vi "Extract maximum.vi"(8 "error in (no error)":errorcluster, 11 "Image in":T1) -> (0 "error out":errorcluster, 1 "Max value":dbl, 2 "y translation":dbl, 3 "x translation":dbl)   [LabVIEW 2012]
uses:
  <vilib>/vision/Image Controls.llb/IMAQ Image.ctl
  <vilib>/vision/NI_Vision_Development_Module.lvlib
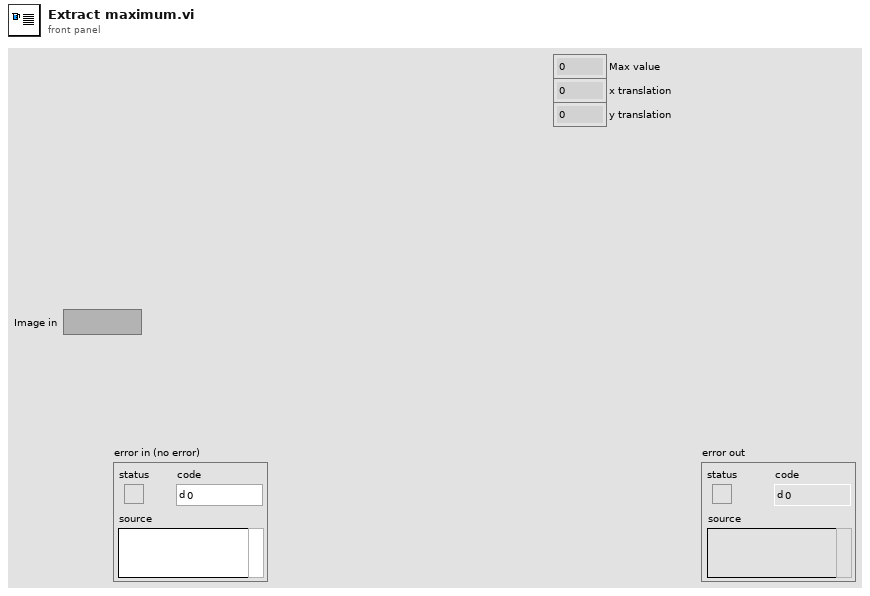
[diagram p1: front panel]
types:
  T1 = typedef "IMAQ Image.ctl" = refnum<image>
  T2 = cluster{"Mean Value":sgl, "Standard Variation":sgl, "Minimal Value":sgl, "Maximal Value":sgl, "Area (calibrated)":sgl, "Area (pixels)":u32, "%":sgl, "Calibration Valid":bool}
  T3 = cluster{"Area":dbl, "Number of Holes":dbl, "Bounding Rect":cluster{"Left":dbl, "Top":dbl, "Right":dbl, "Bottom":dbl}, "Center of Mass":cluster{"X":dbl, "Y":dbl}, "Orientation":dbl, "Dimensions":cluster{"Width":dbl, "Height":dbl}}[]
  T4 = cluster{"Area":dbl, "Number of Holes":dbl, "Bounding Rect":cluster{"Left":dbl, "Top":dbl, "Right":dbl, "Bottom":dbl}, "Center of Mass":cluster{"X":dbl, "Y":dbl}, "Orientation":dbl, "Dimensions":cluster{"Width":dbl, "Height":dbl}}
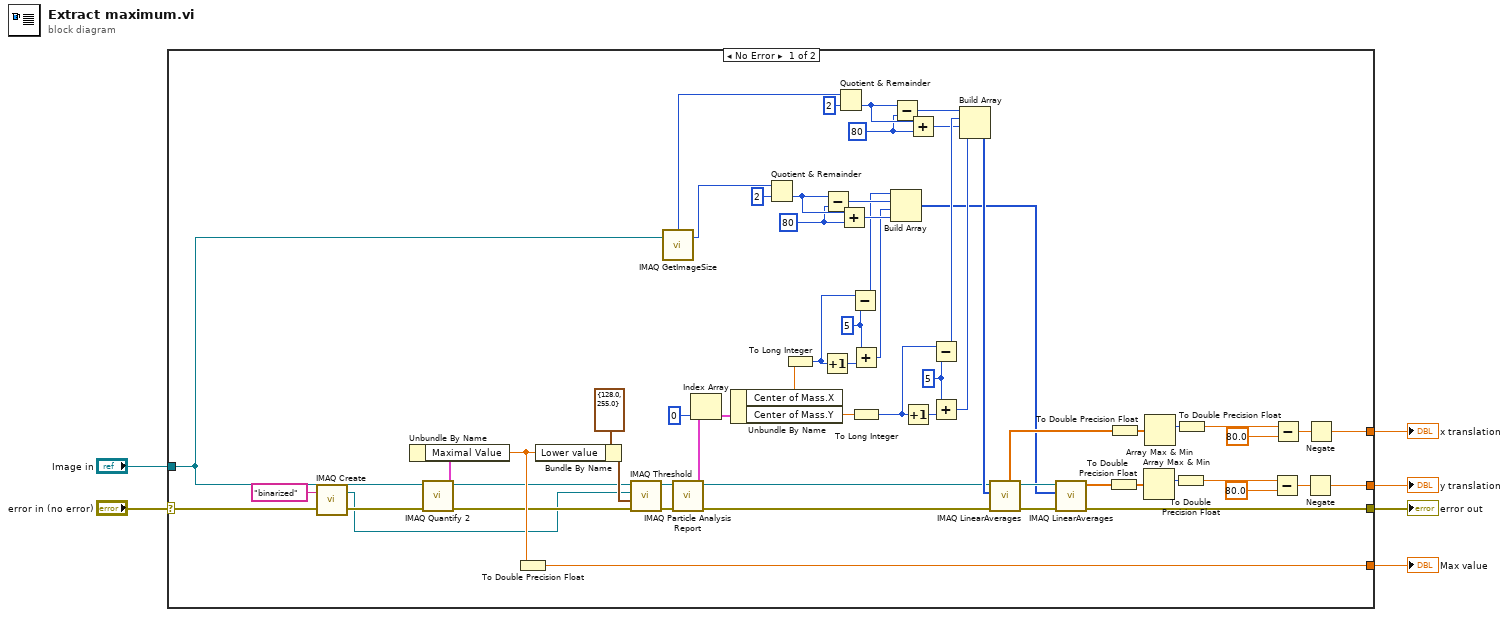
[diagram p0: block diagram]
diagram:
  n1 = case shown="No Error" "error in (no error)" {
    selector: "error in (no error)" -> [w9 w66]
    tunnel: [w12 w66] -> w5
    tunnel: "Image in" -> [w14 _]
    tunnel: [w23 _] -> w3
    tunnel: [w22 _] -> w2
    tunnel: [w11 _] -> w1
    frame No Error {
      w31 = 5 ("y")
      w34 = 80 ("y")
      w42 = 80 ("y")
      w55 = 5 ("y")
      n2 = call "IMAQ Create"("Image Name"="binarized", "error in (no error)"=w9) -> ("New Image"=w7:T1, "error out"=w8:errorcluster)  [unwired: 3 in]
      n3 = call "IMAQ Quantify 2"("error in (no error)"=w8, "Image"=w14) -> ("error out"=w63:errorcluster, "Global Report"=w64:T2)  [unwired: 7 in, 1 out]
      n4 = Unbundle By Name(w64) -> ("Maximal Value"=w65:sgl)
      n5 = To Double Precision Float(number=w65) -> (double precision float=w23:dbl)
      n6 = Bundle By Name(cluster=cluster{"Lower value":sgl, "Upper value":sgl} {"Lower value"=128.0, "Upper value"=255.0} ("Range"), "Lower value"=w65) -> (w61:cluster{"Lower value":sgl, "Upper value":sgl})
      n7 = call "IMAQ Threshold"("error in (no error)"=w63, "Range"=w61, "Image Dst"=w7, "Image Src"=w14) -> ("error out"=w60:errorcluster, "Image Dst Out"=w56:T1)  [unwired: 6 in]
      n8 = call "IMAQ GetImageSize"("Image"=w14) -> ("Y Resolution"=w33:i32, "X Resolution"=w45:i32)  [unwired: 3 in, 1 out]
      n9 = call "IMAQ Particle Analysis Report"("error in (no error)"=w60, "Image"=w56) -> ("error out"=w24:errorcluster, "Particle Reports (Pixels)"=w57:T3)  [unwired: 4 in, 4 out]
      n10 = Index Array(array=w57, index=0) -> (element=w58:T4)
      n11 = Unbundle By Name(w58) -> ("Center of Mass.X"=w32:dbl, "Center of Mass.Y"=w47:dbl)
      n12 = Quotient & Remainder(x=w33, y=2) -> (floor(x/y)=w35:i32)  [unwired: 1 out]
      n13 = To Long Integer(number=w32) -> (32bit integer=w29:i32)
      n14 = Increment(x=w29) -> (x+1=w30:i32)
      n15 = Subtract(x=w35, y=w34) -> (x-y=w28:i32)
      n16 = Quotient & Remainder(x=w45, y=2) -> (floor(x/y)=w43:i32)  [unwired: 1 out]
      n17 = Add(x=w35, y=w34) -> (x+y=w27:i32)
      n18 = Subtract(x=w29, y=w31) -> (x-y=w26:i32)
      n19 = Add(x=w31, y=w30) -> (x+y=w25:i32)
      n20 = To Long Integer(number=w47) -> (32bit integer=w48:i32)
      n21 = Build Array(w26, w28, w25, w27) -> (w13:i32[])
      n22 = Subtract(x=w43, y=w42) -> (x-y=w41:i32)
      n23 = Increment(x=w48) -> (x+1=w44:i32)
      n24 = Add(x=w43, y=w42) -> (x+y=w40:i32)
      n25 = Subtract(x=w48, y=w55) -> (x-y=w51:i32)
      n26 = Add(x=w55, y=w44) -> (x+y=w50:i32)
      n27 = Build Array(w41, w51, w40, w50) -> (w54:i32[])
      n28 = call "IMAQ LinearAverages"("error in (no error)"=w24, "Optional Rectangle"=w54, "Image Src"=w14) -> ("error out"=w15:errorcluster, "X Axis Averages"=w49:sgl[])  [unwired: 4 in, 3 out]
      n29 = call "IMAQ LinearAverages"("error in (no error)"=w15, "Optional Rectangle"=w13, "Image Src"=w14) -> ("error out"=w12:errorcluster, "Y Axis Averages"=w16:sgl[])  [unwired: 4 in, 3 out]
      n30 = To Double Precision Float(number=w16) -> (double precision float=w20:dbl[])
      n31 = To Double Precision Float(number=w49) -> (double precision float=w52:dbl[])
      n32 = Array Max & Min(array=w20) -> (max index (indices)=w21:i32)  [unwired: 3 out]
      n33 = Array Max & Min(array=w52) -> (max index (indices)=w53:i32)  [unwired: 3 out]
      n34 = To Double Precision Float(number=w21) -> (double precision float=w17:dbl)
      n35 = To Double Precision Float(number=w53) -> (double precision float=w37:dbl)
      n36 = Subtract(x=w17, y=80.0) -> (x-y=w18:dbl)
      n37 = Subtract(x=w37, y=80.0) -> (x-y=w38:dbl)
      n38 = Negate(x=w18) -> (-x=w11:dbl)
      n39 = Negate(x=w38) -> (-x=w22:dbl)
    }
    frame Error {
    }
  }
  "error out" <- w5
  "Max value" <- w3
  "x translation" <- w2
  "y translation" <- w1
